vi "Shut Down RT Driver.vi"(11 "RT State Variables in":T1) -> (0 "error out":errorcluster, 3 "RT State Variables out":T1)   [LabVIEW 2019, in "HLA Custom Device Engine.lvlib"]
uses:
  HLA Custom Device Engine.lvlib
  RTStateVariables.ctl
  <vilib>/NI/NIVS Inline Async API/_VS Inline Async API/VS Inline Async API/VS Inline Async API.lvclass
  Shared/Compiled.Settings.ctl
  Shared/main_page_config.ctl
  Shared/object_managament_config.ctl
  Shared/interaction_parameter_configuration.ctl
  Shared/object_attribute_configuration.ctl
  Shared/object_status_info.ctl
  RTruntimeData.ctl
  _typedefs/RThlaMapHelpers.ctl
  _typedefs/map_interaction.ctl
  _typedefs/map_interaction_value.ctl
  _typedefs/map_attr_param_data.ctl
  _typedefs/map_object.ctl
  _typedefs/map_object_key.ctl
  _typedefs/map_object_value.ctl
  _typedefs/map_object_instance.ctl
  _typedefs/map_object_instance_value.ctl
  _typedefs/map_object_vs_instance.ctl
  emea-ni-adg-hla-lv/src/library/typedefs/receiveInteractionEvent_type.ctl
  emea-ni-adg-hla-lv/src/library/typedefs/OrderType.ctl
  emea-ni-adg-hla-lv/src/library/typedefs/TransportationType.ctl
  emea-ni-adg-hla-lv/src/library/typedefs/reflectAttributeValuesEvent_type.ctl
  emea-ni-adg-hla-lv/src/library/typedefs/discoverObjectInstanceEvent_type.ctl
  emea-ni-adg-hla-lv/src/library/typedefs/removeObjectInstanceEvent_type.ctl
  emea-ni-adg-hla-lv/src/library/typedefs/ResignAction.ctl
  emea-ni-adg-hla-lv/src/library/openrti_rti1516eLv.lvlib
  emea-ni-adg-hla-lv/src/helpers/Attribute Handle Set/ahs.lvlib
  emea-ni-adg-hla-lv/src/helpers/Attribute Handle Value Map/ahvm.lvlib
  emea-ni-adg-hla-lv/src/helpers/Parameter Handle Value Map/phvm.lvlib
  Shared/HLA Custom Device Shared.lvlib
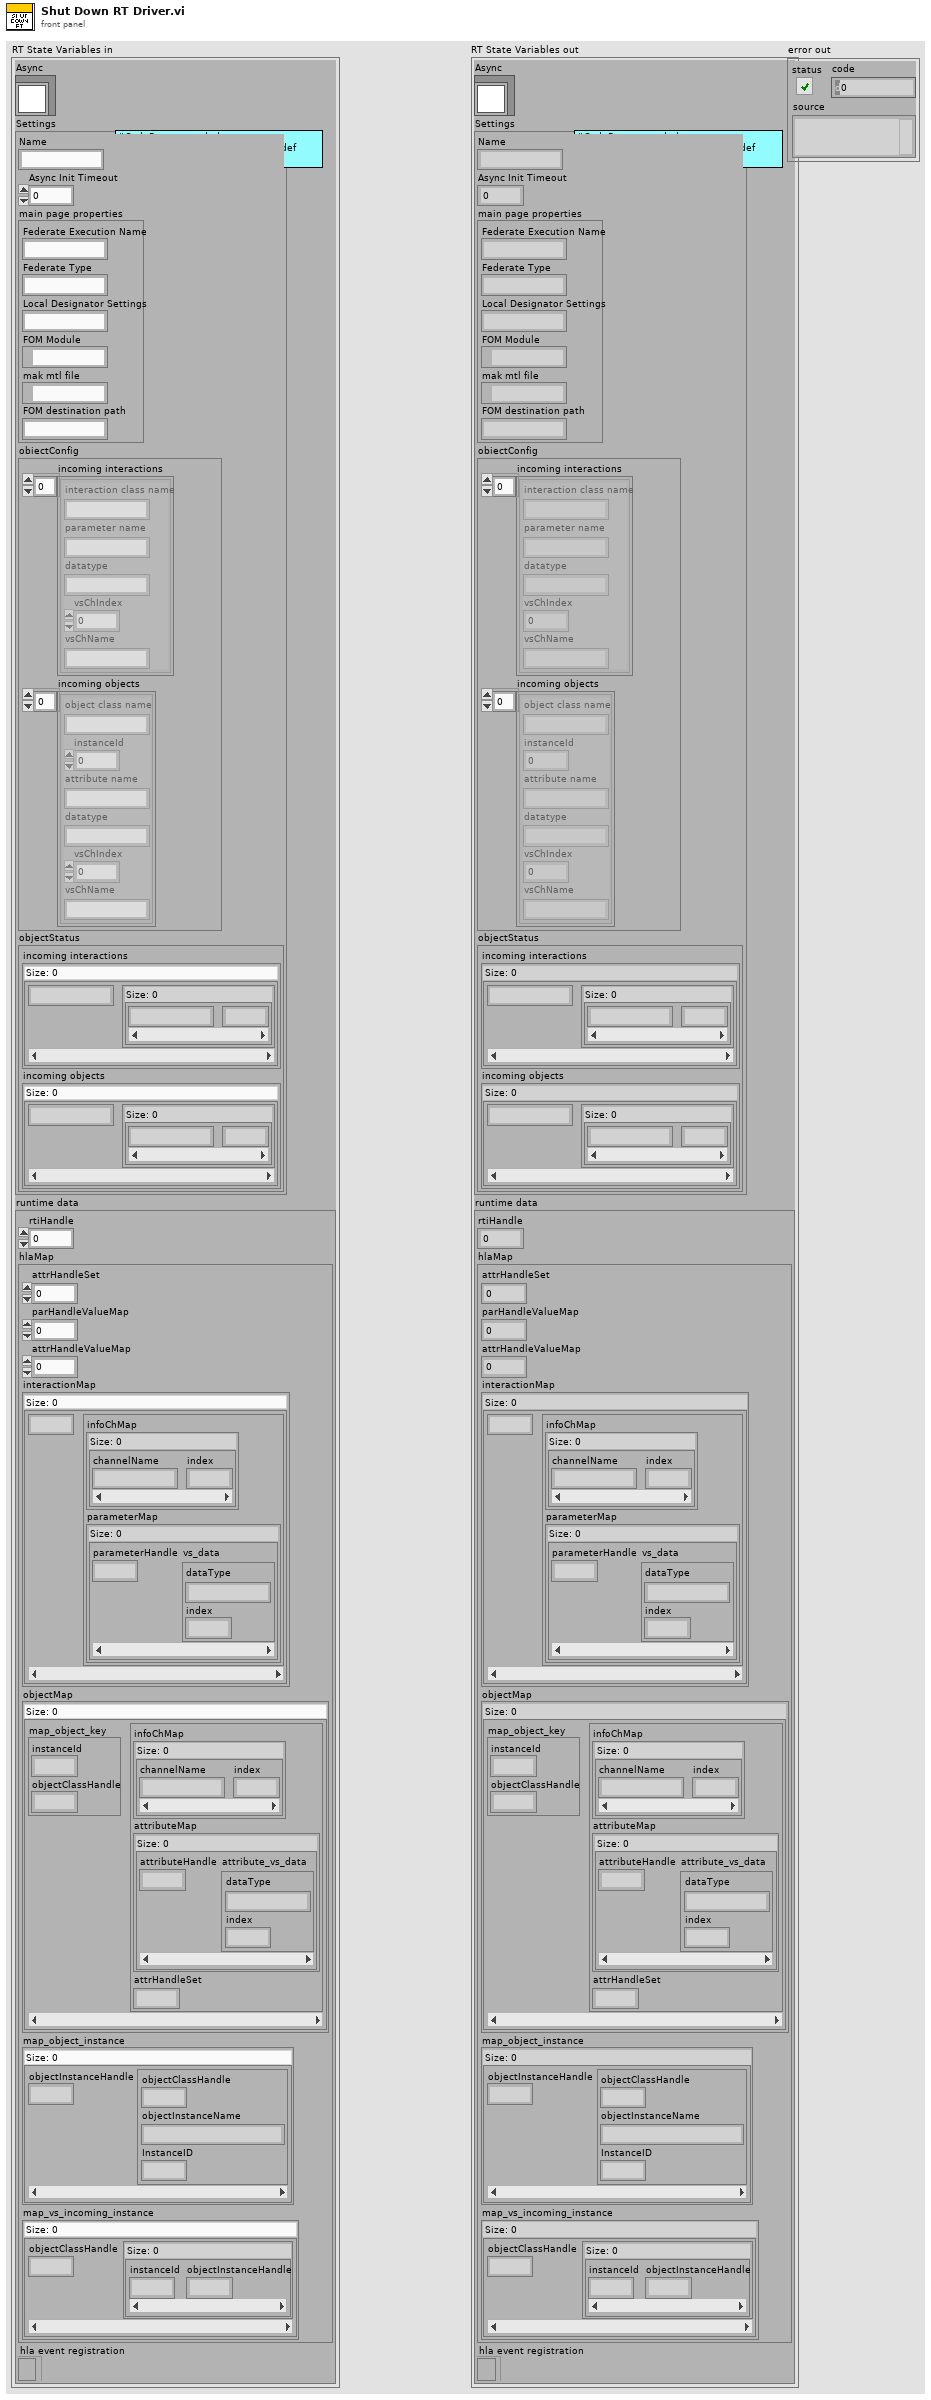
[diagram p1: front panel]
types:
  T1 = typedef "HLA Custom Device Engine.lvlib/RTStateVariables.ctl" = cluster{"Async":refnum<class "VS Inline Async API.lvclass">, "Settings":T2, "runtime data":T8}
  T2 = typedef "HLA Custom Device Shared.lvlib/Compiled.Settings.ctl" = cluster{"Name":string, "Async Init Timeout":u16, "main page properties":T3, "obiectConfig":T4, "objectStatus":T7}
  T3 = typedef "HLA Custom Device Shared.lvlib/main_page_config.ctl" = cluster{"Federate Execution Name":string, "Federate Type":string, "Local Designator Settings":string, "FOM Module":path, "mak mtl file":path, "FOM destination path":string}
  T4 = typedef "HLA Custom Device Shared.lvlib/object_managament_config.ctl" = cluster{"incoming interactions":T5[], "incoming objects":T6[]}
  T5 = typedef "HLA Custom Device Shared.lvlib/interaction_parameter_configuration.ctl" = cluster{"interaction class name":string, "parameter name":string, "datatype":string, "vsChIndex":i32, "vsChName":string}
  T6 = typedef "HLA Custom Device Shared.lvlib/object_attribute_configuration.ctl" = cluster{"object class name":string, "instanceId":i32, "attribute name":string, "datatype":string, "vsChIndex":i32, "vsChName":string}
  T7 = typedef "HLA Custom Device Shared.lvlib/object_status_info.ctl" = cluster{"incoming interactions":map{string, map{string, i32}}, "incoming objects":map{string, map{string, i32}}}
  T8 = typedef "HLA Custom Device Engine.lvlib/RTruntimeData.ctl" = cluster{"rtiHandle":i64, "hlaMap":T9, "hla event registration":refnum<event-registration>}
  T9 = typedef "HLA Custom Device Engine.lvlib/RThlaMapHelpers.ctl" = cluster{"attrHandleSet":u64, "parHandleValueMap":u64, "attrHandleValueMap":u64, "interactionMap":T10, "objectMap":T13, "map_object_instance":T16, "map_vs_incoming_instance":T18}
  T10 = typedef "HLA Custom Device Engine.lvlib/map_interaction.ctl" = map{u64, T11}
  T11 = typedef "HLA Custom Device Engine.lvlib/map_interaction_value.ctl" = cluster{"infoChMap":map{string, i32}, "parameterMap":map{u64, T12}}
  T12 = typedef "HLA Custom Device Engine.lvlib/map_attr_param_data.ctl" = cluster{"dataType":string, "index":i32}
  T13 = typedef "HLA Custom Device Engine.lvlib/map_object.ctl" = map{T14, T15}
  T14 = typedef "HLA Custom Device Engine.lvlib/map_object_key.ctl" = cluster{"instanceId":i32, "objectClassHandle":u64}
  T15 = typedef "HLA Custom Device Engine.lvlib/map_object_value.ctl" = cluster{"infoChMap":map{string, i32}, "attributeMap":map{u64, T12}, "attrHandleSet":u64}
  T16 = typedef "HLA Custom Device Engine.lvlib/map_object_instance.ctl" = map{u64, T17}
  T17 = typedef "HLA Custom Device Engine.lvlib/map_object_instance_value.ctl" = cluster{"objectClassHandle":u64, "objectInstanceName":string, "InstanceID":i32}
  T18 = typedef "HLA Custom Device Engine.lvlib/map_object_vs_instance.ctl" = map{u64, map{i32, u64}}
  T19 = typedef "openrti_rti1516eLv.lvlib/ResignAction.ctl" = enum32{"UNCONDITIONALLY_DIVEST_ATTRIBUTES", "DELETE_OBJECTS", "CANCEL_PENDING_OWNERSHIP_ACQUISITIONS", "DELETE_OBJECTS_THEN_DIVEST", "CANCEL_THEN_DELETE_THEN_DIVEST", "NO_ACTION"}
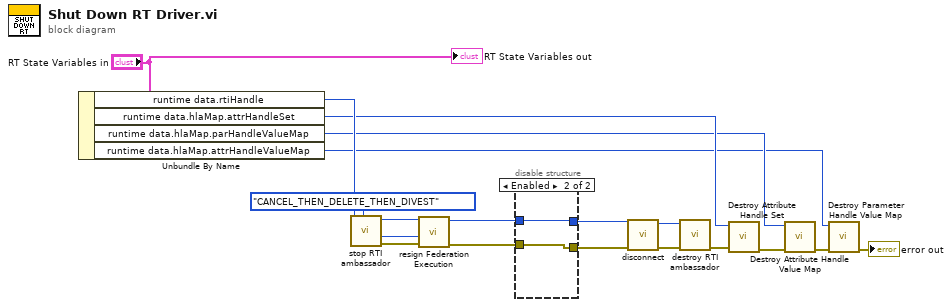
[diagram p0: block diagram]
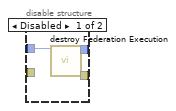
[diagram p2: hidden frame]
diagram:
  n1 = Unbundle By Name("RT State Variables in") -> ("runtime data.rtiHandle"=w5:i64, "runtime data.hlaMap.attrHandleSet"=w4:u64, "runtime data.hlaMap.parHandleValueMap"=w3:u64, "runtime data.hlaMap.attrHandleValueMap"=w2:u64)
  n2 = call "stop RTI ambassador.vi"("rtiHandle in"=w5) -> ("error out"=w12:errorcluster, "rtiHandle out"=w13:i64)  [unwired: 9 in]
  n3 = call "resign Federation Execution.vi"("error in"=w12, "ResignAction(Cancel,Divest)"=ResignAction."CANCEL_THEN_DELETE_THEN_DIVEST", "rtiHandle in"=w13) -> ("error out"=w7:errorcluster, "rtiHandle out"=w10:i64)  [unwired: 7 in]
  n4 = disable-structure "Diagram Disable Structure" shown="Enabled" {
    disable-tunnel: w10 -> [w20 w22]
    disable-tunnel: [w19 w22] -> w9
    disable-tunnel: [_ w21] -> w8
    disable-tunnel: w7 -> [_ w21]
    frame Disabled {
      n5 = call "destroy Federation Execution.vi"("rtiHandle in"=w20) -> ("rtiHandle out"=w19:i64)  [unwired: 9 in, 1 out]
    }
    frame Enabled {
    }
  }
  n6 = call "disconnect.vi"("error in"=w8, "rtiHandle in"=w9) -> ("error out"=w15:errorcluster, "rtiHandle out"=w14:i64)  [unwired: 8 in]
  n7 = call "destroy RTI ambassador.vi"("error in"=w15, "rtiHandle in"=w14) -> ("error out"=w18:errorcluster)  [unwired: 9 in]
  n8 = call "Destroy Attribute Handle Set.vi"("error in"=w18, "attrHandleSet"=w4) -> ("error out"=w17:errorcluster)  [unwired: 8 in, 1 out]
  n9 = call "Destroy Attribute Handle Value Map.vi"("error in"=w17, "attrHandleValueMap in"=w3) -> ("error out"=w16:errorcluster)  [unwired: 8 in, 1 out]
  n10 = call "Destroy Parameter Handle Value Map.vi"("error in"=w16, "attrHandleValueMap in"=w2) -> ("error out"=→"error out":errorcluster)  [unwired: 8 in, 1 out]
  "RT State Variables out" <- "RT State Variables in"
